vi "Simulation Interface.vi"   [LabVIEW 2012]
doc: "[Covers: SI2]"
uses:
  TypeDefs/Simulated Database Command.ctl
  TypeDefs/Error Classification.ctl
types:
  T1 = enum16{"Init", "Handle", "Check", "Close", "Set Current Account"}
  T2 = typedef "Error Classification.ctl" = enum16{"Minor", "Session", "System"}
  T3 = typedef "Simulated Database Command.ctl" = enum16{"Init", "Look up and Lock Account", "Modify Balance", "Get Record", "Commit Record", "Unlock Record", "Close"}
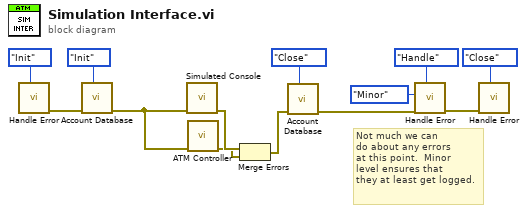
[diagram p0: block diagram]
diagram:
  # "Not much we can\ndo about any errors\nat this point.  Minor\nlevel ensures that\nthey at least get logged."
  n1 = call "Handle Error.vi"("Command"=T1."Init") -> ("error out"=w6:errorcluster)  [unwired: 8 in, 2 out]
  n2 = call "Account Database.vi"("Command"=Simulated_Database_Command."Init", "error in (no error)"=w6) -> ("error out"=w11:errorcluster)  [unwired: 7 in, 2 out]
  n3 = call "Simulated Console.vi"("error in (no error)"=w11) -> ("error out"=w10:errorcluster)  [unwired: 10 in]
  n4 = call "ATM Controller.vi"("error in (no error)"=w11) -> ("error out"=w9:errorcluster)  [unwired: 10 in]
  n5 = Merge Errors(w10, w9) -> (w8:errorcluster)
  n6 = call "Account Database.vi"("Command"=Simulated_Database_Command."Close", "error in (no error)"=w8) -> ("error out"=w4:errorcluster)  [unwired: 7 in, 2 out]
  n7 = call "Handle Error.vi"("Command"=T1."Handle", "error in (no error)"=w4, "Classification"=Error_Classification."Minor") -> ("error out"=w1:errorcluster)  [unwired: 6 in, 2 out]
  n8 = call "Handle Error.vi"("Command"=T1."Close", "error in (no error)"=w1) -> ()  [unwired: 7 in, 3 out]
